vi "command_send.vi"(1 "Commands":string) -> (0 "Response":string)   [LabVIEW 2012]
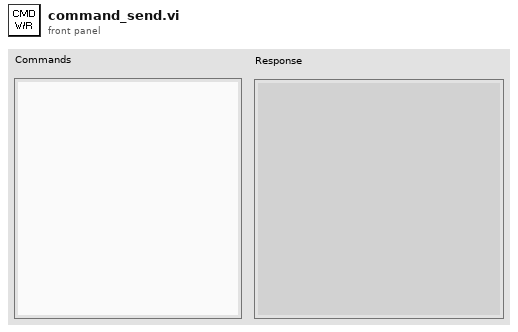
[diagram p1: front panel]
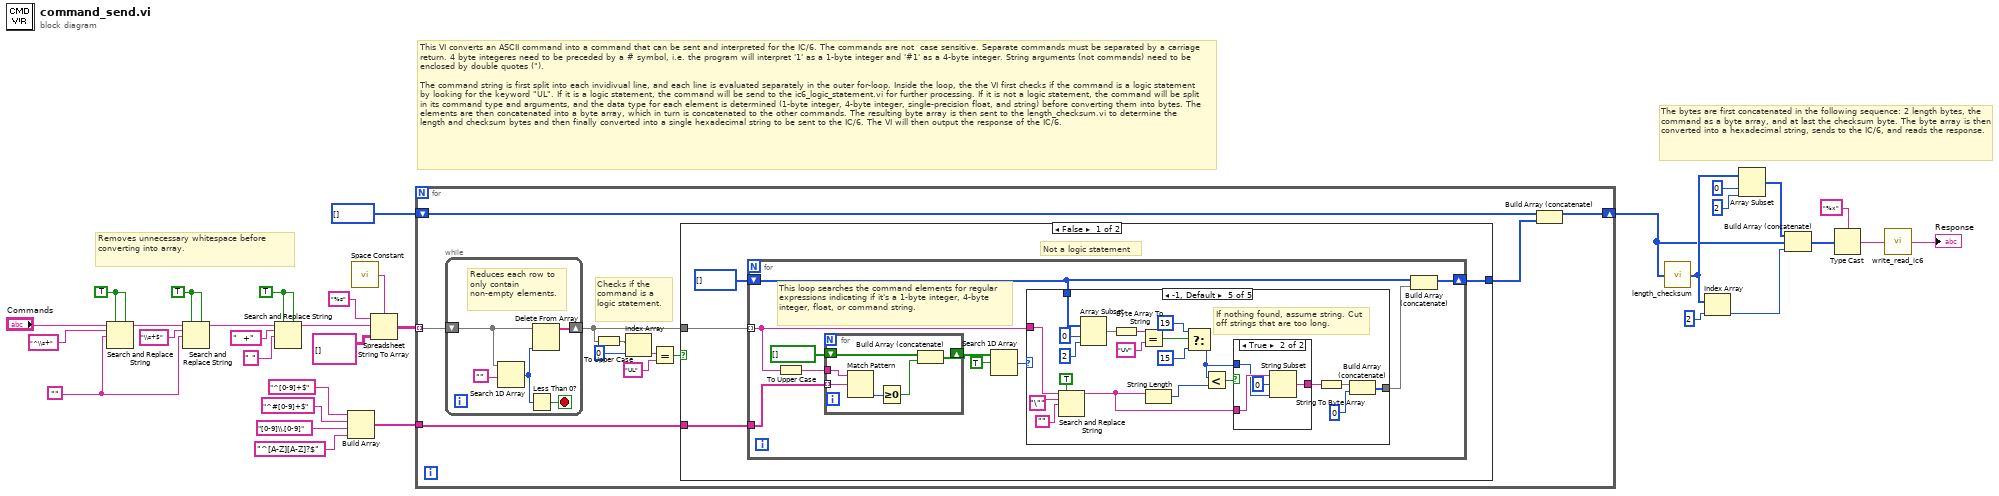
[diagram p0: block diagram]
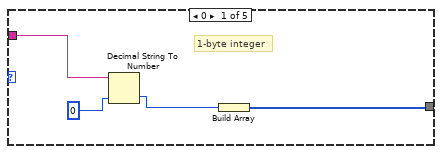
[diagram p2: hidden frame]
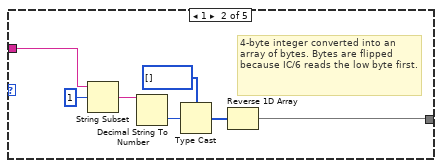
[diagram p3: hidden frame]
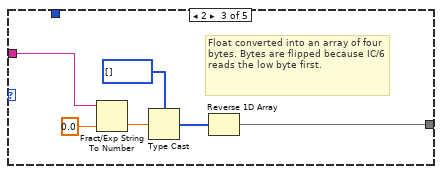
[diagram p4: hidden frame]
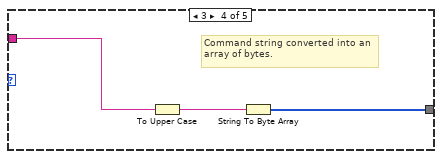
[diagram p5: hidden frame]
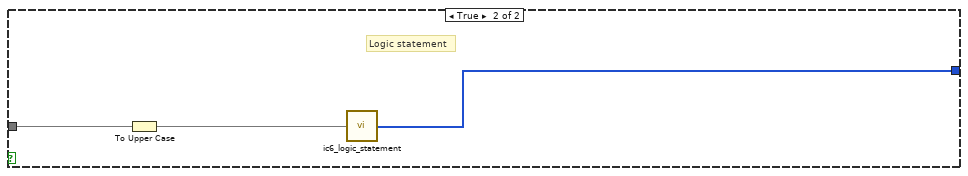
[diagram p7: hidden frame]
diagram:
  w2 = TRUE
  w1 = TRUE
  w4 = ""
  w15 = TRUE
  # "Removes unnecessary whitespace before converting into array."
  # "This VI converts an ASCII command into a command that can be sent and interpreted for the IC/6. The commands are not  case sensitive. Separate commands must be separated by a carriage return. 4 byte integeres need to be preceded by a # symbol, i.e. the program will interpret '1' as a 1-byte integer and '#1' as a 4-byte integer. String arguments (not commands) need to be enclosed by double quotes (\").\n\nThe command string is first split into each invidivual line, and each line is evaluated separately in the outer for-loop. Inside the loop, the the VI first checks if the command is a logic statement by looking for the keyword \"UL\". If it is a logic statement, the command will be send to the ic6_logic_statement.vi for further processing. If it is not a logic statement, the command will be split in its command type and arguments, and the data type for each element is determined (1-byte integer, 4-byte integer, single-precision float, and string) before converting them into bytes. The elements are then concatenated into a byte array, which in turn is concatenated to the other commands. The resulting byte array is then sent to the length_checksum.vi to determine the length and checksum bytes and then finally converted into a single hexadecimal string to be sent to the IC/6. The VI will then output the response of the IC/6."
  # "The bytes are first concatenated in the following sequence: 2 length bytes, the command as a byte array, and at last the checksum byte. The byte array is then converted into a hexadecimal string, sends to the IC/6, and reads the response."
  n1 = Search and Replace String(replace all?=w1, multiline?=w1, input string="Commands", search string="^\\s+", replace string=w4) -> (result string=w7:string)  [unwired: 3 in, 3 out]
  n2 = Search and Replace String(replace all?=w2, multiline?=w2, input string=w7, search string="\\s+$", replace string=w4) -> (result string=w8:string)  [unwired: 3 in, 3 out]
  n3 = Search and Replace String(replace all?=w15, multiline?=w15, input string=w8, search string="  +", replace string=" ") -> (result string=w10:string)  [unwired: 3 in, 3 out]
  n4 = Build Array("^[0-9]+$", "^#[0-9]+$", "[0-9]\\.[0-9]", "^[A-Z][A-Z]?$") -> (w30:string[])
  n5 = call <vilib>:"Space Constant.vi"() -> ("String"=w17:string)
  n6 = Spreadsheet String To Array(delimiter (Tab)=w17, format string="%s", spreadsheet string=w10, array type (2D Dbl)=string[][] []) -> (array=w9:string[][])
  n7 = for {
    tunnel: w9 -> [w40] mode=indexing
    tunnel: w30 -> [w44]
    shift-right: [w42] -> w23
    shift-left: u8[] [] -> [w41]
    # "Checks if the command is a logic statement."
    n8 = while {
      shift-right: [w118] -> w34
      shift-left: w40 -> [w114]
      stop <- w116 stop-if-true
      # "Reduces each row to only contain non-empty elements."
      n9 = Search 1D Array(1D array=w114, element="") -> (index of element=w117:i32)  [unwired: 1 in]
      n10 = Less Than 0?(x=w117) -> (x < 0?=w116:bool)
      n11 = Delete From Array(array=w114, index=w117) -> (array with subset deleted=w118:string[])  [unwired: 1 in, 1 out]
    }
    n12 = To Upper Case(1:w34) -> (0:w35:string[])
    n13 = Index Array(array=w35, index=0) -> (element=w37:string)
    n14 = Equal?(x=w37, y="UL") -> (x = y?=w39:bool)
    n15 = case shown="False" w39 {
      tunnel: w44 -> [w48 _]
      tunnel: [w46 w113] -> w43
      tunnel: w34 -> [w45 w112]
      frame False {
        # "Not a logic statement"
        n16 = for {
          tunnel: w45 -> [w55] mode=indexing
          tunnel: w48 -> [w53]
          shift-right: [w52] -> w46
          shift-left: u8[] [] -> [w50]
          # "This loop searches the command elements for regular expressions indicating if it's a 1-byte integer, 4-byte integer, float, or command string."
          n17 = To Upper Case(1:w55) -> (0:w49:string)
          n18 = for {
            tunnel: w49 -> [w110]
            shift-right: [w108] -> w58
            shift-left: bool[] [] -> [w107]
            tunnel: w53 -> [w105] mode=indexing
            n19 = Match Pattern(string=w110, regular expression=w105) -> (offset past match=w106:i32)  [unwired: 1 in, 3 out]
            n20 = Greater Or Equal To 0?(x=w106) -> (x >= 0?=w109:bool)
            n21 = Build Array (concatenate)(w107, w109) -> (w108:bool[])
          }
          n22 = Search 1D Array(1D array=w58, element=TRUE) -> (index of element=w56:i32)  [unwired: 1 in]
          n23 = case shown="-1, Default" w56 {
            tunnel: w55 -> [w62 w64 w71 w78 w87]
            tunnel: [w60 w63 w70 w77 w99] -> w51
            tunnel: w50 -> [_ _ _ _ w96]
            frame 0 {
              # "1-byte integer"
              n24 = Decimal String To Number(string=w62, default (0L)=u8 0) -> (number=w59:u8)  [unwired: 1 in, 1 out]
              n25 = Build Array(w59) -> (w60:u8[])
            }
            frame 1 {
              # "4-byte integer converted into an array of bytes. Bytes are flipped because IC/6 reads the low byte first."
              n26 = String Subset(string=w64, offset (0)=1) -> (substring=w68:string)  [unwired: 1 in]
              n27 = Decimal String To Number(string=w68) -> (number=w67:i32)  [unwired: 2 in, 1 out]
              n28 = Type Cast(type=u8[] [], x=w67) -> (*(type *) &x=w65:u8[])
              n29 = Reverse 1D Array(array=w65) -> (reversed array=w63:u8[])
            }
            frame 2 {
              # "Float converted into an array of four bytes. Bytes are flipped because IC/6 reads the low byte first."
              n30 = Fract/Exp String To Number(string=w71, default (0 dbl)=sgl 0.0) -> (number=w75:sgl)  [unwired: 2 in, 1 out]
              n31 = Type Cast(type=u8[] [], x=w75) -> (*(type *) &x=w74:u8[])
              n32 = Reverse 1D Array(array=w74) -> (reversed array=w70:u8[])
            }
            frame 3 {
              # "Command string converted into an array of bytes."
              n33 = To Upper Case(1:w78) -> (0:w76:string)
              n34 = String To Byte Array(string=w76) -> (unsigned byte array=w77:u8[])
            }
            frame -1, Default {
              # "If nothing found, assume string. Cut off strings that are too long."
              n35 = Search and Replace String(replace all?=TRUE, input string=w87, search string="\"", replace string="") -> (result string=w79:string)  [unwired: 4 in, 3 out]
              n36 = Array Subset(array=w96, index=0, length=2) -> (w93:u8[])
              n37 = Byte Array To String(unsigned byte array=w93) -> (string=w92:string)
              n38 = Equal?(x=w92, y="UV") -> (x = y?=w83:bool)
              n39 = String Length(string=w79) -> (length=w81:i32)
              n40 = Select(t=19, s=w83, f=15) -> (s? t:f=w80:i32)
              n41 = Less?(x=w80, y=w81) -> (x < y?=w82:bool)
              n42 = case shown="True" w82 {
                tunnel: [w100 w104] -> w86
                tunnel: w80 -> [_ w102]
                tunnel: w79 -> [w100 w103]
                frame False {
                }
                frame True {
                  n43 = String Subset(string=w103, offset (0)=0, length (rest)=w102) -> (substring=w104:string)
                }
              }
              n44 = String To Byte Array(string=w86) -> (unsigned byte array=w97:u8[])
              n45 = Build Array (concatenate)(w97, u8 0) -> (w99:u8[])
            }
          }
          n46 = Build Array (concatenate)(w50, w51) -> (w52:u8[])
        }
      }
      frame True {
        # "Logic statement"
        n47 = To Upper Case(1:w112) -> (0:w111:string[])
        n48 = call "ic6_logic_statement.vi"("Logic statement"=w111) -> ("Byte output"=w113:u8[])
      }
    }
    n49 = Build Array (concatenate)(w41, w43) -> (w42:u8[])
  }
  n50 = call "length_checksum.vi"("Input Byte Array"=w23) -> ("Size byte + checksum"=w24:u8[])
  n51 = Index Array(array=w24, index=2) -> (element=w28:u8)
  n52 = Array Subset(array=w24, index=0, length=2) -> (w22:u8[])
  n53 = Build Array (concatenate)(w22, w23, w28) -> (w21:u8[])
  n54 = Type Cast(type="%x", x=w21) -> (*(type *) &x=w12:string)
  n55 = call "write_read_ic6.vi"("Input string"=w12) -> ("Output string"=→"Response":string)
